vi "Write Filter Bandwidth.vi"(8 "error in (no error)":errorcluster, 10 "Filter Bandwidth":dbl(knob)=5.0 scale=0.0..1.0, 11 "HRF_Device in":refnum<class "HRF_Device.lvclass">) -> (0 "error out":errorcluster, 3 "HRF_Device out":refnum<class "HRF_Device.lvclass">)   [LabVIEW 2020, in "HRF_Device.lvclass"]
uses:
  HRF_Device.lvclass
  HRF_Device.lvclass/HRF_Device.ctl
  D:/work/HackRF/Labview Driver/NetHackrf.dll
  NetHackrf.dll
  Read Device ref.vi
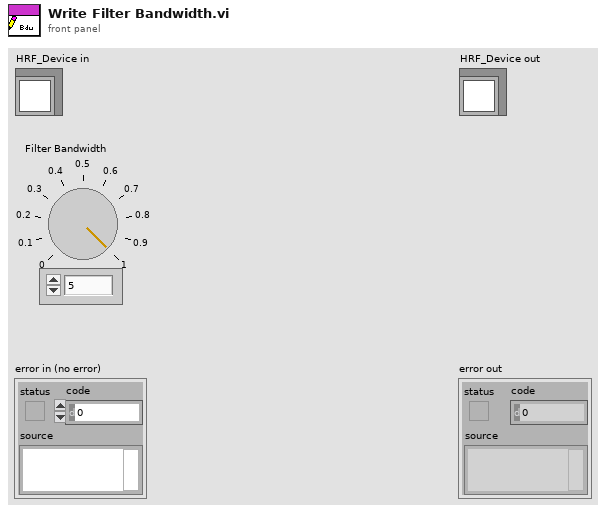
[diagram p1: front panel]
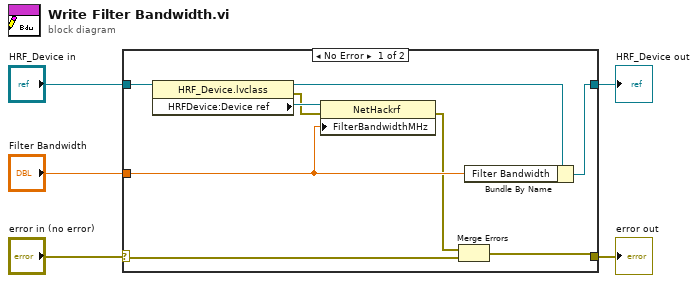
[diagram p0: block diagram]
diagram:
  n1 = case shown="No Error" "error in (no error)" {
    selector: "error in (no error)" -> [w8 w15]
    tunnel: [w7 w15] -> w4
    tunnel: [w13 w16] -> w2
    tunnel: "HRF_Device in" -> [w14 w16]
    tunnel: "Filter Bandwidth" -> [w10 _]
    frame No Error {
      n2 = property class="HRF_Device.lvclass"(reference=w14) -> (reference out=w12:refnum<class "HRF_Device.lvclass">, error out=w9:errorcluster, "HRFDevice:Device ref"=w11:refnum<k24>)  [unwired: 1 in]
      n3 = property class="NetHackrf"(reference=w11, error in=w9, "FilterBandwidthMHz"=w10) -> (error out=w6:errorcluster)  [unwired: 1 out]
      n4 = Merge Errors(w6, w8) -> (w7:errorcluster)
      n5 = Bundle By Name(cluster=w12, "Filter Bandwidth"=w10) -> (w13:refnum<class "HRF_Device.lvclass">)
    }
    frame Error {
    }
  }
  "error out" <- w4
  "HRF_Device out" <- w2
